vi "Uniquify Execution Unit Name.vi"(7 "custom device ref":T1=18446744073709551615 format="%.0x", 10 "execution unit name":string) -> (2 "execution unit name out":string)   [LabVIEW 2020, in "AIM ARINC 664 Engine.lvlib" / "Implementation.lvlib" / "Execution Unit Factory.lvclass"]
uses:
  Execution Unit Factory.lvclass
  <vilib>/NI VeriStand/Custom Device API/Custom Device Item Ref.ctl
  Execution Unit Factory.lvclass/Execution Unit Factory.ctl
  <vilib>/NI VeriStand/Custom Device API/Custom Device API.lvlib
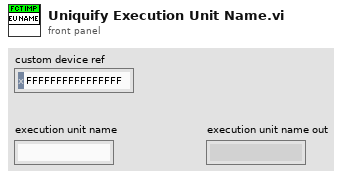
[diagram p1: front panel]
types:
  T1 = typedef "Custom Device API.lvlib/Custom Device Item Ref.ctl" = u64
  T2 = typedef "Custom Device API.lvlib/Custom Device Item Info.ctl" = cluster{"Name":string, "Is Channel":bool, "GUID":string, "Is Waveform":bool}
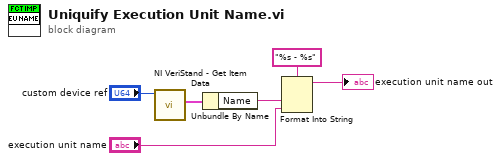
[diagram p0: block diagram]
diagram:
  n1 = call <vilib>:"NI VeriStand - Get Item Data.vi"("Item Ref in"="custom device ref") -> ("Item Info"=w6:T2)  [unwired: 7 in, 3 out]
  n2 = Unbundle By Name(w6) -> ("Name"=w4:string)
  n3 = Format Into String(format string="%s - %s", w4, "execution unit name") -> (resulting string=→"execution unit name out":string)  [unwired: 2 in, 1 out]
